vi "Create Message Getter (from Template).vi"(8 "error in (no error)":errorcluster, 10 "RPC Message Name":string, 11 "RPC Messages Folder (ProjectItem) in":refnum<vi>) -> (0 "error out":errorcluster, 1 "Created?":bool, 2 "Getter VI out":refnum<vi>, 3 "RPC Messages Folder (ProjectItem) out":refnum<vi>)   [LabVIEW 2019, in "gRPC Scripting Tools.lvlib"]
uses:
  gRPC Scripting Tools.lvlib
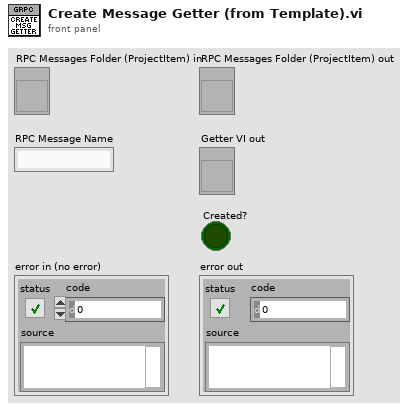
[diagram p1: front panel]
types:
  T1 = enum32{"invalid VI type", "Standard VI", "Control VI", "Global VI", "Polymorphic VI", "Configuration VI", "SubSystem", "Facade VI", "Method VI"}
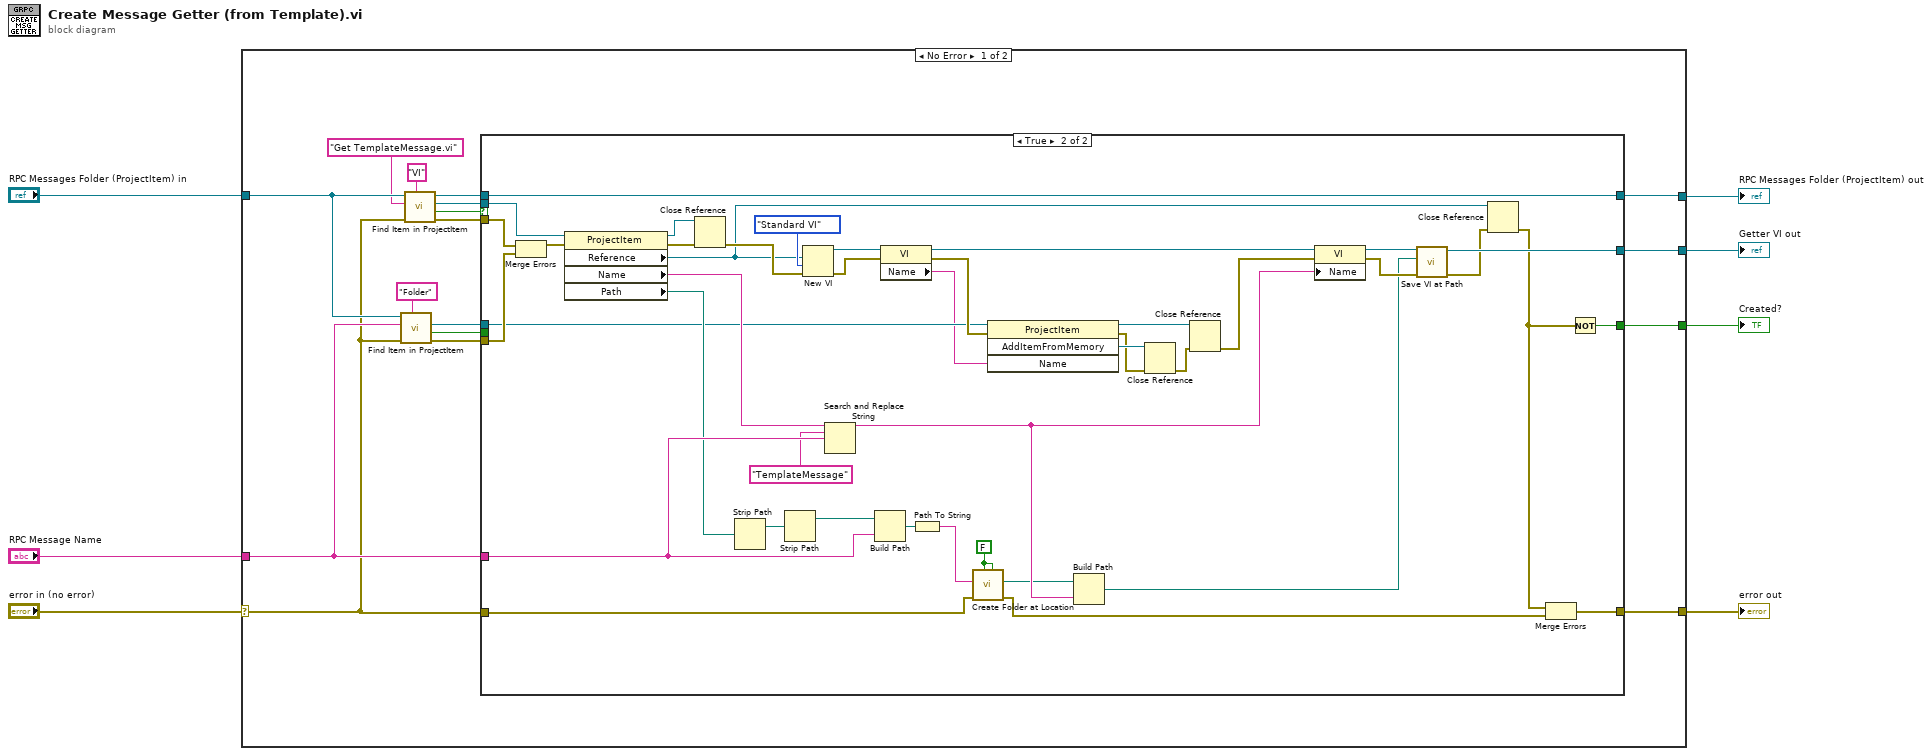
[diagram p0: block diagram]
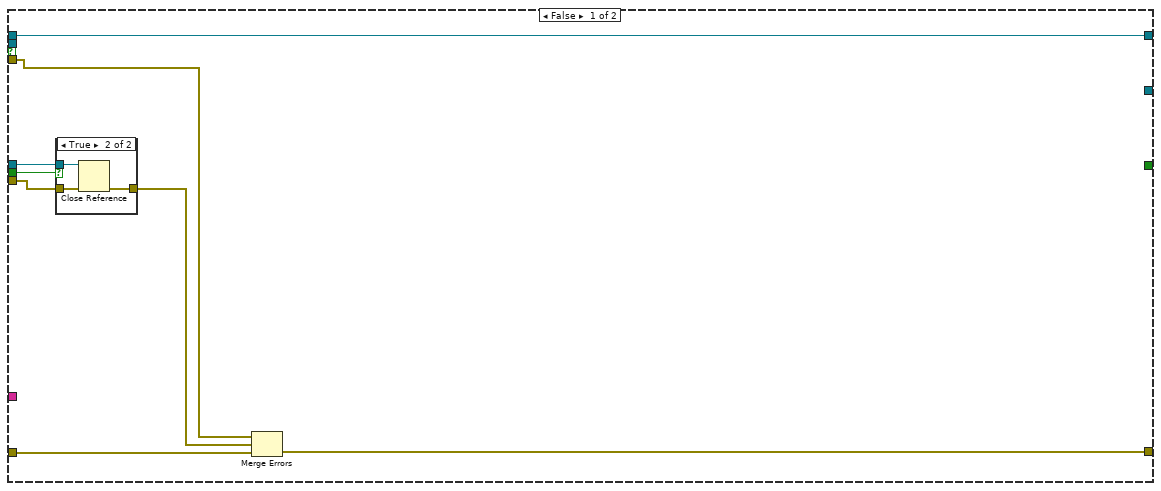
[diagram p2: hidden frame]
diagram:
  n1 = case shown="No Error" "error in (no error)" {
    selector: "error in (no error)" -> [w13 w79]
    tunnel: "RPC Message Name" -> [w24 _]
    tunnel: "RPC Messages Folder (ProjectItem) in" -> [w23 w80]
    tunnel: [w22 w79] -> w5
    tunnel: [w10 w80] -> w4
    tunnel: [w19 _] -> w3
    tunnel: [w9 _] -> w1
    frame No Error {
      n2 = call "Find Item in ProjectItem.vi"("Item Type"="Folder", "error in (no error)"=w13, "Name"=w24, "ProjectItem in"=w23) -> ("error out"=w21:errorcluster, "Found ?"=w8:bool, "Item Refnum out"=w18:refnum<vi>)  [unwired: 4 in, 1 out]
      n3 = call "Find Item in ProjectItem.vi"("Item Type"="VI", "error in (no error)"=w13, "Name"="Get TemplateMessage.vi", "ProjectItem in"=w23) -> ("error out"=w20:errorcluster, "Found ?"=w12:bool, "Item Refnum out"=w17:refnum<vi>, "ProjectItem out"=w11:refnum<vi>)  [unwired: 4 in]
      n4 = case shown="True" w12 {
        tunnel: w24 -> [_ w78]
        tunnel: [w27 w74] -> w22
        tunnel: w21 -> [w31 w72]
        tunnel: w20 -> [w25 w70]
        tunnel: [_ w68] -> w19
        tunnel: w18 -> [w30 w53]
        tunnel: w17 -> [_ w48]
        tunnel: w13 -> [w28 w47]
        tunnel: w11 -> [w32 w46]
        tunnel: [w32 w46] -> w10
        tunnel: [_ w43] -> w9
        tunnel: w8 -> [w26 _]
        frame False {
          n5 = case shown="True" w26 {
            tunnel: w31 -> [w33 w36]
            tunnel: w30 -> [_ w35]
            tunnel: [w33 w34] -> w29
            frame False {
            }
            frame True {
              n6 = Close Reference(reference=w35, error in (no error)=w36) -> (error out=w34:errorcluster)
            }
          }
          n7 = Merge Errors(w25, w29, w28) -> (w27:errorcluster)
        }
        frame True {
          w69 = FALSE ("Use Relative (F)")
          n8 = Merge Errors(w70, w72) -> (w71:errorcluster)
          n9 = property class="ProjectItem"(reference=w48, error in=w71) -> (reference out=w77:refnum<vi>, error out=w75:errorcluster, "Reference"=w37:refnum<vi>, "Name"=w60:string, "Path"=w58:path)
          n10 = Close Reference(reference=w77, error in (no error)=w75) -> (error out=w76:errorcluster)
          n11 = Strip Path(path=w58) -> (stripped path=w54:path)  [unwired: 1 out]
          n12 = Strip Path(path=w54) -> (stripped path=w55:path)  [unwired: 1 out]
          n13 = New VI(8:w76, 9:T1."Standard VI" ("vi type (standard vi)"), 10:w37) -> (0:w51:errorcluster, 3:w49:refnum<vi>)  [unwired: 1 in, 3 out]
          n14 = Search and Replace String(input string=w60, search string="TemplateMessage", replace string=w78) -> (result string=w64:string)  [unwired: 5 in, 3 out]
          n15 = Build Path(base path=w55, name or relative path=w78) -> (appended path=w56:path)
          n16 = property class="VI"(reference=w49, error in=w51) -> (reference out=w61:refnum<vi>, error out=w62:errorcluster, "Name"=w52:string)
          n17 = Path To String(path=w56) -> (string=w57:string)
          n18 = call "Create Folder at Location.vi"("Override existing (F)"=w69, "Use Relative (F)"=w69, "Error In"=w47, "Path"=w57) -> ("Error Out"=w73:errorcluster, "Full path out"=w63:path)  [unwired: 5 in, 1 out]
          n19 = invoke class="ProjectItem" method="AddItemFromMemory"(reference=w53, error in=w62, "Name"=w52) -> (reference out=w45:refnum<vi>, error out=w41:errorcluster, "AddItemFromMemory"=w42:refnum<vi>)  [unwired: 1 in, 1 out]
          n20 = Build Path(base path=w63, name or relative path=w64) -> (appended path=w66:path)
          n21 = Close Reference(reference=w42, error in (no error)=w41) -> (error out=w40:errorcluster)
          n22 = Close Reference(reference=w45, error in (no error)=w40) -> (error out=w44:errorcluster)
          n23 = property class="VI"(reference=w61, error in=w44, "Name"=w64) -> (reference out=w65:refnum<vi>, error out=w67:errorcluster)
          n24 = call "Save VI at Path.vi"("error in (no error)"=w67, "Path"=w66, "VI in"=w65) -> ("error out"=w39:errorcluster, "VI out"=w68:refnum<vi>)  [unwired: 6 in, 1 out]
          n25 = Close Reference(reference=w37, error in (no error)=w39) -> (error out=w38:errorcluster)
          n26 = Merge Errors(w38, w73) -> (w74:errorcluster)
          n27 = Not(x=w38) -> (.not. x?=w43:bool)
        }
      }
    }
    frame Error {
    }
  }
  "error out" <- w5
  "RPC Messages Folder (ProjectItem) out" <- w4
  "Getter VI out" <- w3
  "Created?" <- w1
